vi "8q_conflict.vi"(9 "nextX":i32, 11 "State":i32[](array[numeric])=[1, 3]) -> (3 "Available":bool)   [LabVIEW 2012]
panel:
  out "i":i32
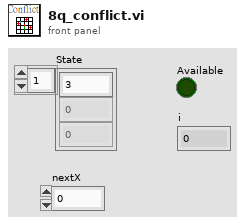
[diagram p1: front panel]
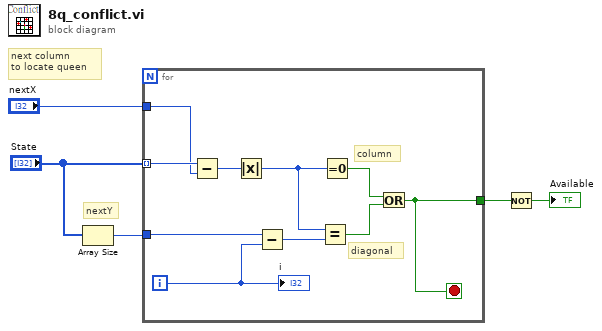
[diagram p0: block diagram]
diagram:
  # "next column \nto locate queen"
  # "nextY"
  n1 = Array Size(array="State") -> (size(s)=w4:i32)
  n2 = for {
    tunnel: "State" -> [w15] mode=indexing
    tunnel: w4 -> [w11]
    tunnel: "nextX" -> [w14]
    tunnel: [w6] -> w1
    i -> [w12]
    stop <- w6 stop-if-true
    # "diagonal"
    # "column"
    n3 = Subtract(x=w15, y=w14) -> (x-y=w13:i32)
    n4 = Absolute Value(x=w13) -> (abs(x)=w9:i32)
    n5 = Subtract(x=w11, y=w12) -> (x-y=w10:i32)
    n6 = Equal?(x=w9, y=w10) -> (x = y?=w7:bool)
    n7 = Equal To 0?(x=w9) -> (x = 0?=w8:bool)
    n8 = Or(x=w8, y=w7) -> (x .or. y?=w6:bool)
    "i" <- w12
  }
  n9 = Not(x=w1) -> (.not. x?=→"Available":bool)
